vi "Set Extension.vi"(8 "error in (no error)":errorcluster, 11 "TDMS Report":refnum<class "TDMS Report - Solution.lvclass">) -> (0 "error out":errorcluster, 3 "TDMS Report out":refnum<class "TDMS Report - Solution.lvclass">)   [LabVIEW 2011, in "TDMS Report - Solution.lvclass"]
doc: "Part of the solution for the TDMS Report Object. This is a dynamic dispatch VI that overrides the associated method in the parent.\n\nAAL 9/09"
uses:
  TDMS Report - Solution.lvclass
  Report Class/Report.lvclass
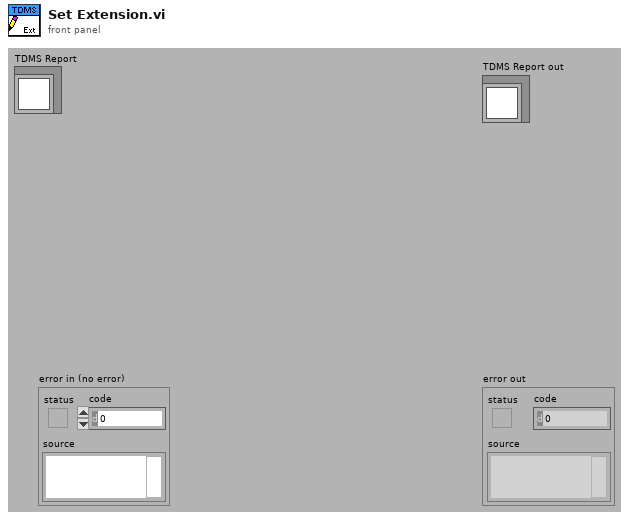
[diagram p1: front panel]
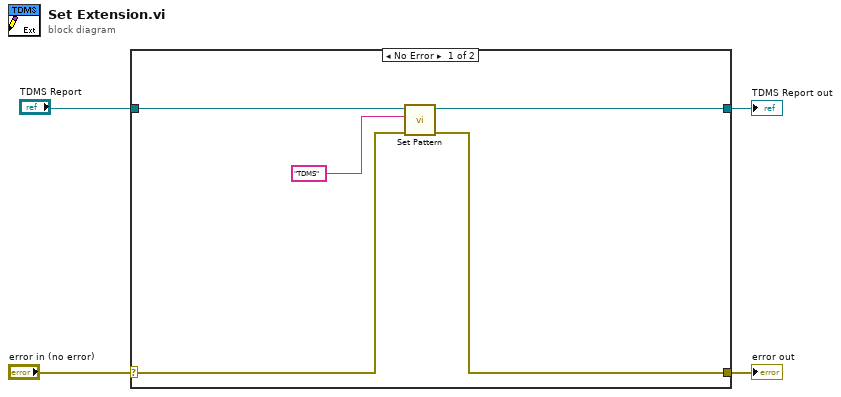
[diagram p0: block diagram]
diagram:
  n1 = case shown="No Error" "error in (no error)" {
    selector: "error in (no error)" -> [w7 w11]
    tunnel: [w6 w11] -> w3
    tunnel: [w9 w10] -> w2
    tunnel: "TDMS Report" -> [w5 w10]
    frame No Error {
      n2 = call "Set Pattern.vi"("error in (no error)"=w7, "Pattern"="TDMS", "Report"=w5) -> ("error out"=w6:errorcluster, "Report out"=w9:refnum<class "TDMS Report - Solution.lvclass">)  [unwired: 7 out]
    }
    frame Error {
    }
  }
  "error out" <- w3
  "TDMS Report out" <- w2
